vi "Convert (g,s,f) to (tf, tm).vi"(6 "IRF offset":dbl[unit] format="%#.3e", 9 "Phasor Harmonic Frequency":dbl[unit], 10 "Phasor (g, s)":T1) -> (1 "Modulus Lifetime":dbl[unit] format="%#.3e", 2 "Phase Lifetime":dbl[unit] format="%#.3e")   [LabVIEW 2019]
uses:
  Phasor (g, s).ctl
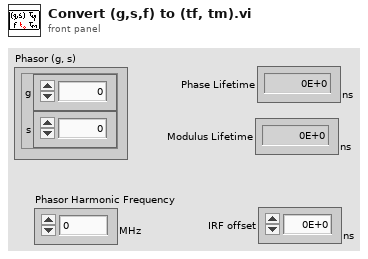
[diagram p1: front panel]
types:
  T1 = typedef "Phasor (g, s).ctl" = cluster{"g":dbl, "s":dbl}
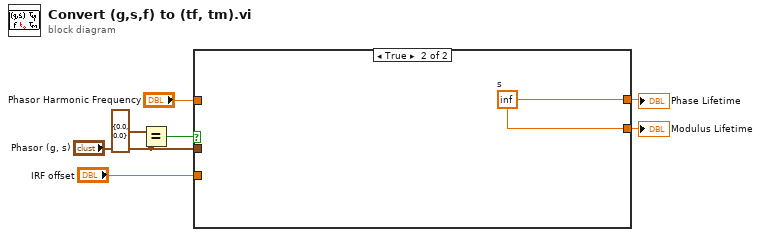
[diagram p0: block diagram]
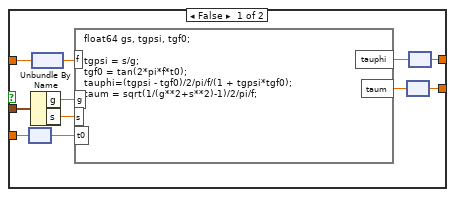
[diagram p2: hidden frame]
diagram:
  n1 = Equal?(x=T1 {"g"=0.0, "s"=0.0}, y="Phasor (g, s)") -> (x = y?=w1:bool)
  n2 = case shown="True" w1 {
    tunnel: "Phasor Harmonic Frequency" -> [w14 _]
    tunnel: [w12 w19] -> w6
    tunnel: [w11 w19] -> w5
    tunnel: "IRF offset" -> [w10 _]
    tunnel: "Phasor (g, s)" -> [w8 _]
    frame False {
      n3 = node(w10) -> (w9:dbl)
      n4 = Unbundle By Name(w8) -> ("g"=w17:dbl, "s"=w18:dbl)
      n5 = node(w14) -> (w13:dbl)
      n6 = formula code="float64 gs, tgpsi, tgf0;\n\ntgpsi = s/g;\ntgf0 = tan(2*pi*f*t0);\ntauphi=(tgpsi - tgf0)/2/pi/f/(1 + tgpsi*tgf0);\ntaum = sqrt(1/(g**2+s**2)-1)/2/pi/f;"("f"=w13, "g"=w17, "s"=w18, "t0"=w9) -> ("tauphi"=w15:dbl, "taum"=w16:dbl)
      n7 = node(w16) -> (w11:dbl[unit])
      n8 = node(w15) -> (w12:dbl[unit])
    }
    frame True {
      w19 = dbl[unit] inf  # s
    }
  }
  "Phase Lifetime" <- w6
  "Modulus Lifetime" <- w5
